vi "Test_Flip_ARGB.vi"(8 "error in (no error)":errorcluster, 11 "Test Case In":refnum<class "Image.lvclass">) -> (0 "error out":errorcluster, 3 "Test Case Out":refnum<class "Image.lvclass">)   [LabVIEW 2020, in "g_ar_toolkit.test.lvlib" / "Image.lvclass"]
uses:
  Image.lvclass
  Image.lvclass/Image.ctl
  g_ar_toolkit.image/g_ar_toolkit.image.lvlib
  g_ar_toolkit.image/Image Size (Fixed).ctl
  g_ar_toolkit.image/CreateEmptyImageARGB.vi
  g_ar_toolkit.image/FlipARGB.vi
  g_ar_toolkit.image/Flip Mode.ctl
  4993e8ee-a06a-463a-9684-69129f64d5ce.vi
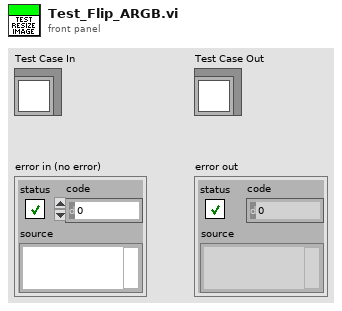
[diagram p1: front panel]
types:
  T1 = typedef "g_ar_toolkit.image.lvlib/Flip Mode.ctl" = enum16{"X-Axis", "Y-Axis", "X and Y Axes"}
  T2 = typedef "g_ar_toolkit.image.lvlib/Image Size (Fixed).ctl" = cluster{"Width":u16, "Height":u16}
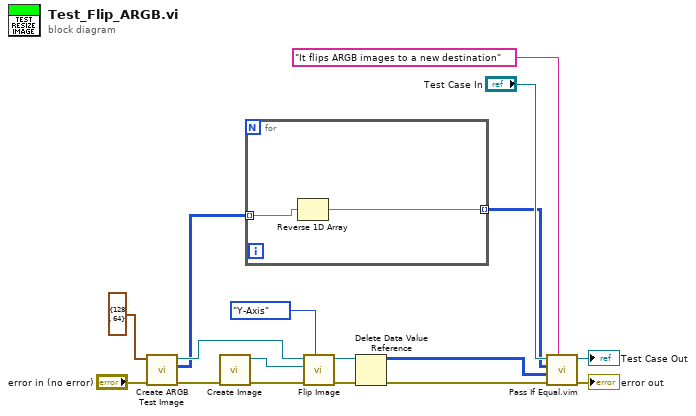
[diagram p0: block diagram]
diagram:
  n1 = call "Create ARGB Test Image.vi"("error in (no error)"="error in (no error)", "Preallocated Image Size"=T2 {"Width"=128, "Height"=64} ("Preallocated Image Size (Default - 0,0)")) -> ("error out"=w3:errorcluster, "24-bit pixmap"=w4:u32[][], "Data Value Reference out"=w5:refnum<data-value>)  [unwired: 7 in]
  n2 = call-poly "Create Image.vi"("error in (no error)"=w3) -> ("error out"=w9:errorcluster, "New ARGB Image"=w7:refnum<data-value>)  [unwired: 9 in]
  n3 = for {
    tunnel: w4 -> [w19] mode=indexing
    tunnel: [w18] -> w2 mode=indexing
    n4 = Reverse 1D Array(array=w19) -> (reversed array=w18:u32[])
  }
  n5 = call-poly "Flip Image.vi"("Flip Mode (Default: Y-Axis)"=Flip_Mode."Y-Axis" ("Flip Mode (Default: X-Axis)"), "error in (no error)"=w9, "ARGB Destination Image"=w7, "ARGB Source Image"=w5) -> ("error out"=w11:errorcluster, "ARGB  Destination Image (duplicate)"=w12:refnum<data-value>)  [unwired: 6 in]
  n6 = Delete Data Value Reference(data value reference=w12, error in=w11) -> (data value=w8:u32[][], error out=w14:errorcluster)
  n7 = call "Pass If Equal.vim"("Description"="It flips ARGB images to a new destination", "error in (no error)"=w14, "Actual"=w8, "Expected"=w2, "LUnit Test Case In"="Test Case In") -> ("error out"=→"error out":errorcluster, "LUnit Test Case Out"=→"Test Case Out":refnum<class "Image.lvclass">)  [unwired: 5 in]
